vi "MT_Close.vi"(8 "Error In":errorcluster caption="错误输入") -> (0 "Error Out":errorcluster caption="错误输出")   [LabVIEW 2020]
uses:
  lib/MT/MT_API.lvlib
panel:
  # "关闭MT设备"
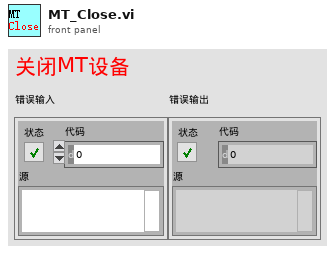
[diagram p1: front panel]
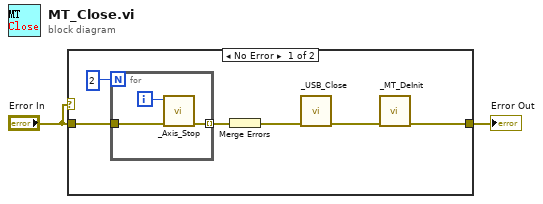
[diagram p0: block diagram]
diagram:
  n1 = case shown="No Error" "Error In" {
    tunnel: [w7 w12] -> w2
    tunnel: "Error In" -> [w5 w12]
    frame No Error {
      n2 = for {
        N: 2 -> [_]
        tunnel: w5 -> [w10]
        tunnel: [w9] -> w4 mode=indexing
        i -> [w11]
        n3 = call "_Axis_Stop.vi"("Error In"=w10, "轴序号"=w11) -> ("Error Out"=w9:errorcluster)  [unwired: 9 in]
      }
      n4 = Merge Errors(w4) -> (w3:errorcluster)
      n5 = call "_USB_Close.vi"("Error In"=w3) -> ("Error Out"=w8:errorcluster)  [unwired: 10 in]
      n6 = call "_MT_DeInit.vi"("Error In"=w8) -> ("Error Out"=w7:errorcluster)  [unwired: 10 in]
    }
    frame Error {
    }
  }
  "Error Out" <- w2
